vi "Normalize.vi"(8 "error in (no error)":errorcluster, 10 "eval":dbl, 11 "TestObjetive in":refnum<class "TestObjetive.lvclass">) -> (0 "error out":errorcluster, 2 "normalizedEval":dbl, 3 "TestObjetive out":refnum<class "TestObjetive.lvclass">)   [LabVIEW 2023, in "TestObjetive.lvclass"]
uses:
  TestObjetive.lvclass
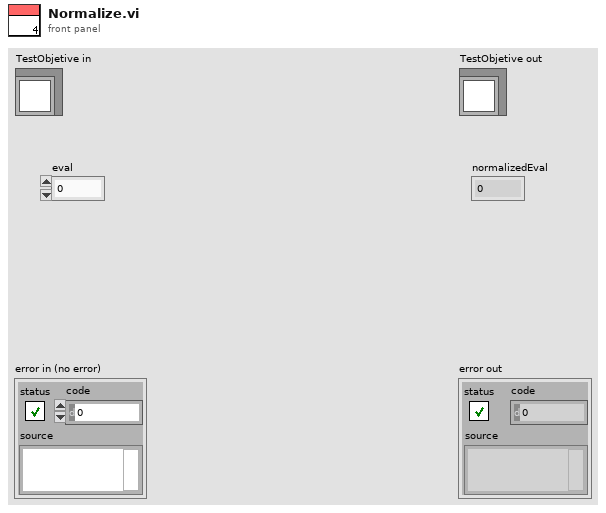
[diagram p1: front panel]
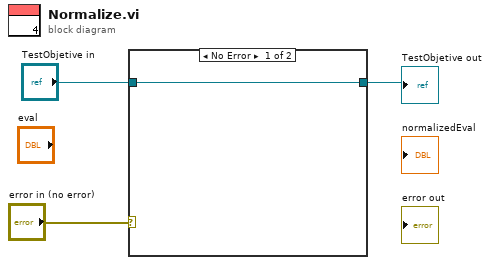
[diagram p0: block diagram]
diagram:
  n1 = case shown="No Error" "error in (no error)" {
    tunnel: "TestObjetive in" -> [w4 w5]
    tunnel: [w4 w5] -> w1
    frame No Error {
    }
    frame Error {
    }
  }
  "TestObjetive out" <- w1
